vi "PAUSE_RAND.vi"() -> ()   [LabVIEW 2015]
uses:
  Global.vi
  oskar_tools/oskar_tools.lvlib
panel:
  out "timed out":bool
  in  "timeout (ms)":u32=30000
  out "iteration":i32
  out "Random":dbl=0.48554270802337385
  in  "Rec":string="PRAND"
  in  "stop":bool
  out "VAR index":i32
  out "Var value":u32=2000
  out "Old_Value":u32=2000
  out "Set":bool=TRUE
  out "Recieved":bool=TRUE
  in  "Var":string="PAUSE"
  # "Wait (ms) and record a random number.\n\nValue Type: U32\nOptions: none"
  # "Debug"
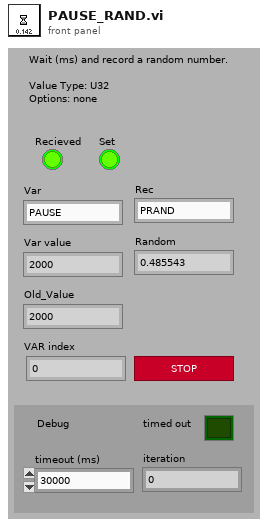
[diagram p1: front panel]
types:
  T1 = typedef "Semaphore RefNum" = refnum<k1>
  T2 = cluster{"VAR":string, "Options":string, "Val":string, "Recieved":bool, "Set":bool}[]
  T3 = cluster{"VAR":string, "Options":string, "Val":string, "Recieved":bool, "Set":bool}
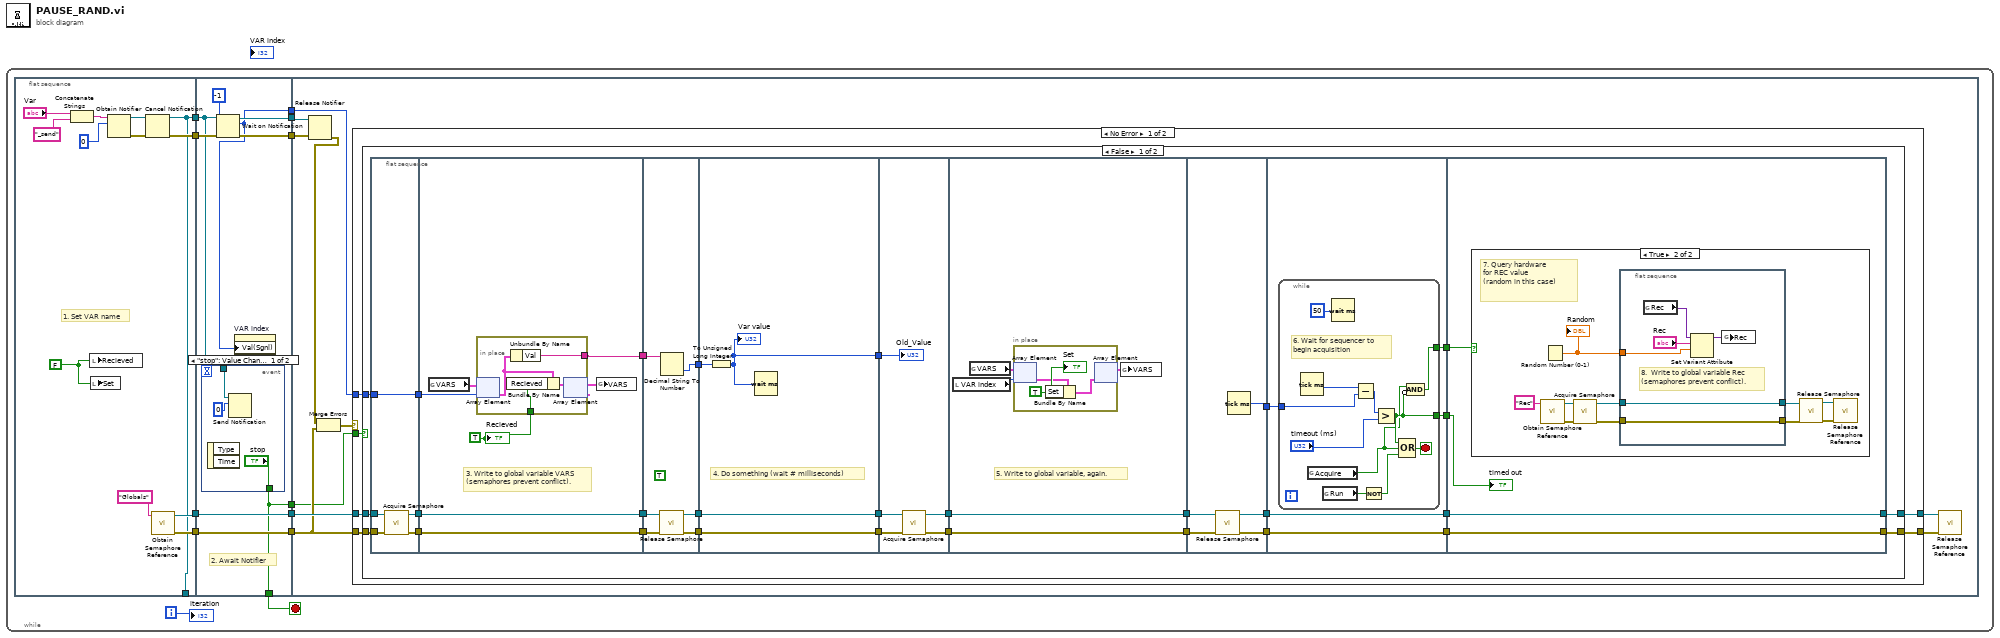
[diagram p0: block diagram]
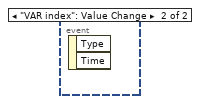
[diagram p2: hidden frame]
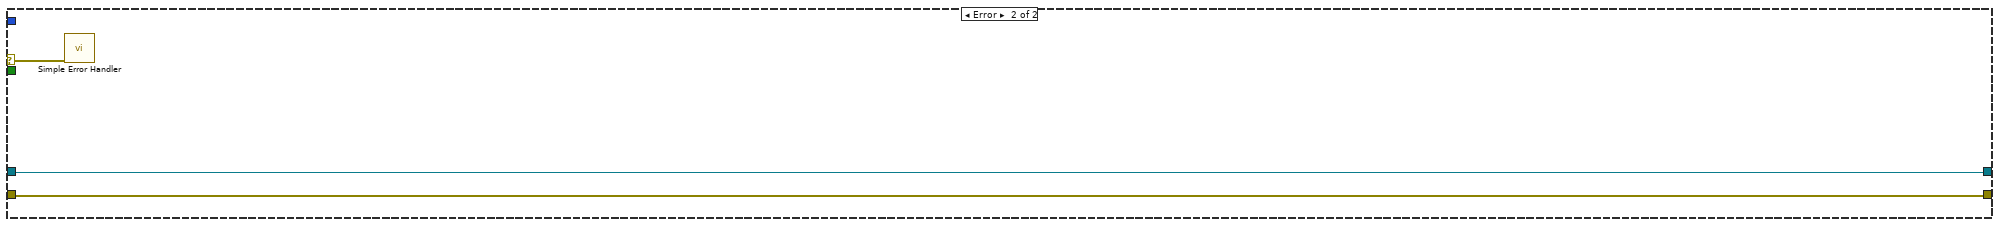
[diagram p5: hidden frame]
diagram:
  n1 = while {
    i -> [w1]
    stop <- w3 stop-if-true
    n2 = flat-sequence {
      tunnel: [w15] -> w12
      tunnel: [w14] -> w11
      tunnel: [w22] -> w7
      tunnel: [w21] -> w5
      tunnel: [w14] -> _
      tunnel: w12 -> [w32]
      tunnel: w11 -> [w26]
      tunnel: [w31] -> w10
      tunnel: [w28] -> w9
      tunnel: [w27] -> w8
      tunnel: w7 -> [w30]
      tunnel: [w30] -> w6
      tunnel: w5 -> [w29]
      tunnel: [w29] -> w4
      tunnel: [w25] -> w3
      tunnel: [w25] -> w2
      tunnel: w10 -> [w39]
      tunnel: w9 -> [w40]
      tunnel: w8 -> [w46]
      tunnel: w6 -> [w45]
      tunnel: w4 -> [w42]
      tunnel: w2 -> [w37]
      frame #0 {
        w24 = FALSE ("notification")
        # "1. Set VAR name"
        n3 = Concatenate Strings("Var", "_send") -> (w19:string)
        n4 = local write "Recieved"(w24) -> ()
        n5 = local write "Set"(w24) -> ()
        n6 = Obtain Notifier(name (unnamed)=w19, notification data type=0) -> (notifier out=w13:refnum<notifier>, error out=w16:errorcluster)  [unwired: 2 in, 1 out]
        n7 = Cancel Notification(0:w13, 3:w16) -> (8:w14:refnum<notifier>, 11:w15:errorcluster)  [unwired: 1 out]
        n8 = call <vilib>:"Obtain Semaphore Reference.vi"("name (unnamed)"="Globals") -> ("error out"=w21:errorcluster, "semaphore"=w22:T1)  [unwired: 4 in, 1 out]
      }
      frame #1 {
        # "2. Await Notifier"
        n9 = event shown="[0] \"stop\": Value Change" {
          selector: _ -> [_ _]
          dyn-events: _ -> [_ _]
          timeout: _ -> [_ _]
          tunnel: ["stop" _] -> w25
          tunnel: w26 -> [w35 _]
          event "stop": Value Change {
            n10 = event-data() -> ()  [unwired: 1 in, 2 out]
            n11 = Send Notification(notification=0, notifier=w35) -> ()  [unwired: 1 in, 2 out]
          }
          event "VAR index": Value Change {
            n12 = event-data() -> ()  [unwired: 1 in, 2 out]
          }
        }
        n13 = Wait on Notification(notifier=w26, timeout in ms (-1)=-1, error in (no error)=w32) -> (notifier out=w31:refnum<notifier>, notification=w27:i32, error out=w28:errorcluster)  [unwired: 1 in, 1 out]
        n14 = property on="VAR index" class="DigNum (strict)"("Val(Sgnl)"=w27) -> ()  [unwired: 2 in, 2 out]
      }
      frame #2 {
        n15 = Release Notifier(notifier=w39, error in (no error)=w40) -> (error out=w38:errorcluster)  [unwired: 1 in, 2 out]
        n16 = Merge Errors(w38, w42) -> (w41:errorcluster)
        n17 = case shown="No Error" w41 {
          selector: w41 -> [_ w163]
          tunnel: w46 -> [w52 _]
          tunnel: w45 -> [w51 w165]
          tunnel: w42 -> [w50 w164]
          tunnel: [w49 w164] -> w44
          tunnel: [w48 w165] -> w43
          tunnel: w37 -> [w47 _]
          frame No Error {
            n18 = case shown="False" w47 {
              tunnel: w52 -> [w65 _]
              tunnel: w51 -> [w64 w162]
              tunnel: w50 -> [w63 w161]
              tunnel: [w62 w161] -> w49
              tunnel: [w61 w162] -> w48
              frame False {
                n19 = flat-sequence {
                  tunnel: w63 -> [w83]
                  tunnel: w64 -> [w84]
                  tunnel: w65 -> [w85]
                  tunnel: [w85] -> w80
                  tunnel: [w82] -> w79
                  tunnel: [w81] -> w78
                  tunnel: w80 -> [w87]
                  tunnel: w79 -> [w91]
                  tunnel: w78 -> [w92]
                  tunnel: [w92] -> w77
                  tunnel: [w91] -> w76
                  tunnel: [w86] -> w75
                  tunnel: w77 -> [w101]
                  tunnel: w76 -> [w102]
                  tunnel: [w100] -> w74
                  tunnel: [w99] -> w73
                  tunnel: [w97] -> w72
                  tunnel: w75 -> [w98]
                  tunnel: w74 -> [w106]
                  tunnel: w73 -> [w105]
                  tunnel: [w106] -> w71
                  tunnel: [w105] -> w70
                  tunnel: w72 -> [w104]
                  tunnel: [w103] -> w60
                  tunnel: w71 -> [w111]
                  tunnel: w70 -> [w108]
                  tunnel: [w110] -> w69
                  tunnel: [w109] -> w68
                  tunnel: w60 -> [w107]
                  tunnel: [w116] -> w67
                  tunnel: w69 -> [w116]
                  tunnel: [w112] -> w66
                  tunnel: w68 -> [w112]
                  tunnel: w67 -> [w124]
                  tunnel: w66 -> [w123]
                  tunnel: [w122] -> w59
                  tunnel: [w121] -> w58
                  tunnel: [w120] -> w55
                  tunnel: w59 -> [w129]
                  tunnel: w58 -> [w128]
                  tunnel: [w129] -> w57
                  tunnel: [w128] -> w56
                  tunnel: w55 -> [w127]
                  tunnel: [w126] -> w54
                  tunnel: [w125] -> w53
                  tunnel: [w143] -> w61
                  tunnel: [w144] -> w62
                  tunnel: w53 -> [w141]
                  tunnel: w54 -> [w142]
                  tunnel: w56 -> [w143]
                  tunnel: w57 -> [w144]
                  frame #0 {
                    n20 = call <vilib>:"Acquire Semaphore.vi"("error in (no error)"=w83, "semaphore"=w84) -> ("error out"=w82:errorcluster, "semaphore out"=w81:T1)  [unwired: 3 in, 1 out]
                  }
                  frame #1 {
                    w88 = TRUE ("Found")
                    # "3. Write to global variable VARS\n(semaphores prevent conflict)."
                    n21 = global read "Global.vi" "VARS"() -> (w89:T2)
                    n22 = in-place {
                      in-place-border: [w94] -> w86
                      in-place-border: w88 -> [w93]
                      n23 = in-place-array #1(w89, w87) -> (w96:T3)
                      n24 = Bundle By Name(cluster=w96, "Recieved"=w93) -> (w95:T3)
                      n25 = Unbundle By Name(w96) -> ("Val"=w94:string)
                      n26 = in-place-array #1(w95) -> (w90:T2)  [unwired: 1 out]
                    }
                    n27 = global write "Global.vi" "VARS"(w90) -> ()
                    "Recieved" <- w88
                  }
                  frame #2 {
                    (unwired) TRUE ("Blinking")
                    n28 = call <vilib>:"Release Semaphore.vi"("error in (no error)"=w102, "semaphore"=w101) -> ("error out"=w99:errorcluster, "semaphore out"=w100:T1)  [unwired: 4 in]
                    n29 = Decimal String To Number(string=w98) -> (number=w97:i32)  [unwired: 2 in, 1 out]
                  }
                  frame #3 {
                    # "4. Do something (wait # milliseconds)"
                    n30 = To Unsigned Long Integer(number=w104) -> (unsigned 32bit integer=w103:u32)
                    "Var value" <- w103
                    n31 = Wait (ms)(milliseconds to wait=w103) -> ()  [unwired: 1 out]
                  }
                  frame #4 {
                    n32 = call <vilib>:"Acquire Semaphore.vi"("error in (no error)"=w108, "semaphore"=w111) -> ("error out"=w109:errorcluster, "semaphore out"=w110:T1)  [unwired: 3 in, 1 out]
                    "Old_Value" <- w107
                  }
                  frame #5 {
                    # "5. Write to global variable, again."
                    n33 = local read "VAR index"() -> (w115:i32)
                    n34 = global read "Global.vi" "VARS"() -> (w114:T2)
                    n35 = in-place {
                      w119 = TRUE ("Set")
                      n36 = in-place-array #2(w114, w115) -> (w118:T3)
                      n37 = Bundle By Name(cluster=w118, "Set"=w119) -> (w117:T3)
                      n38 = in-place-array #2(w117) -> (w113:T2)  [unwired: 1 out]
                      "Set" <- w119
                    }
                    n39 = global write "Global.vi" "VARS"(w113) -> ()
                  }
                  frame #6 {
                    n40 = call <vilib>:"Release Semaphore.vi"("error in (no error)"=w123, "semaphore"=w124) -> ("error out"=w122:errorcluster, "semaphore out"=w121:T1)  [unwired: 4 in]
                    n41 = Tick Count (ms)() -> (millisecond timer value=w120:u32)
                  }
                  frame #7 {
                    n42 = while {
                      tunnel: w127 -> [w138]
                      tunnel: [w132] -> w126
                      tunnel: [w130] -> w125
                      stop <- w135 stop-if-true
                      # "6. Wait for sequencer to \nbegin acquisition"
                      n43 = Tick Count (ms)() -> (millisecond timer value=w139:u32)
                      n44 = global read "Global.vi" "Acquire"() -> (w131:bool)
                      n45 = global read "Global.vi" "Run"() -> (w134:bool)
                      n46 = Wait (ms)(milliseconds to wait=u32 50) -> ()  [unwired: 1 out]
                      n47 = Subtract(x=w139, y=w138) -> (x-y=w137:u32)
                      n48 = Not(x=w134) -> (.not. x?=w133:bool)
                      n49 = Greater?(x=w137, y="timeout (ms)") -> (0:w132:bool)
                      n50 = Compound Arithmetic op=OR(w132, w131, w133) -> (w135:bool)
                      n51 = Compound Arithmetic op=AND(w131, invert w132) -> (w130:bool)
                    }
                  }
                  frame #8 {
                    n52 = case shown="True" w141 {
                      frame False {
                      }
                      frame True {
                        # "7. Query hardware\nfor REC value\n(random in this case)"
                        n53 = call <vilib>:"Obtain Semaphore Reference.vi"("name (unnamed)"="Rec") -> ("error out"=w150:errorcluster, "semaphore"=w154:T1)  [unwired: 4 in, 1 out]
                        n54 = Random Number (0-1)() -> (number: 0 to 1=w149:dbl)
                        "Random" <- w149
                        n55 = call <vilib>:"Acquire Semaphore.vi"("error in (no error)"=w150, "semaphore"=w154) -> ("error out"=w151:errorcluster, "semaphore out"=w152:T1)  [unwired: 3 in, 1 out]
                        n56 = flat-sequence {
                          tunnel: w152 -> [w156]
                          tunnel: w151 -> [w155]
                          tunnel: w149 -> [w157]
                          tunnel: [w156] -> w145
                          tunnel: [w155] -> w146
                          frame #0 {
                            # "8.  Write to global variable Rec\n(semaphores prevent conflict)."
                            n57 = global read "Global.vi" "Rec"() -> (w158:variant)
                            n58 = Set Variant Attribute(Variant=w158, name="Rec", value=w157) -> (Variant out=w159:variant)  [unwired: 1 in, 2 out]
                            n59 = global write "Global.vi" "Rec"(w159) -> ()
                          }
                        }
                        n60 = call <vilib>:"Release Semaphore.vi"("error in (no error)"=w146, "semaphore"=w145) -> ("error out"=w147:errorcluster, "semaphore out"=w148:T1)  [unwired: 4 in]
                        n61 = call <vilib>:"Release Semaphore Reference.vi"("error in (no error)"=w147, "semaphore"=w148) -> ()  [unwired: 8 in, 2 out]
                      }
                    }
                    "timed out" <- w142
                  }
                }
              }
              frame True {
              }
            }
          }
          frame Error {
            n62 = call <vilib>:"Simple Error Handler.vi"("error in (no error)"=w163) -> ()  [unwired: 4 in, 5 out]
          }
        }
        n63 = call <vilib>:"Release Semaphore Reference.vi"("error in (no error)"=w44, "semaphore"=w43) -> ()  [unwired: 8 in, 2 out]
      }
    }
    "iteration" <- w1
  }
